vi "动态调用.vi"() -> ()   [LabVIEW 2011]
panel:
  in  "Stop Button":bool
  in  "Play Button":bool
  out "Gauge":dbl(knob) scale=0.0..10.0
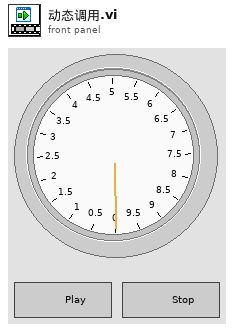
[diagram p1: front panel]
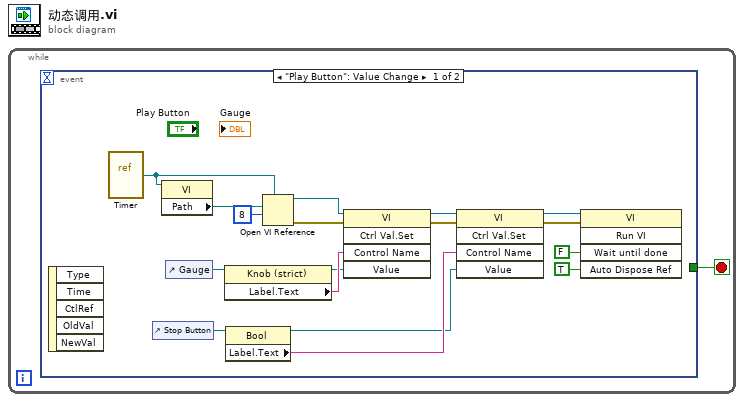
[diagram p0: block diagram]
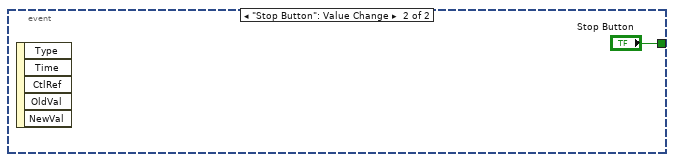
[diagram p2: hidden frame]
diagram:
  n1 = while {
    stop <- w1 stop-if-true
    n2 = event shown="[0] \"Play Button\": Value Change" {
      selector: _ -> [_ _]
      dyn-events: _ -> [_ _]
      timeout: _ -> [_ _]
      tunnel: [_ "Stop Button"] -> w1
      event "Play Button": Value Change {
        n3 = event-data() -> ()  [unwired: 1 in, 5 out]
        n4 = vi-ref "Timer.vi"() -> (w18:refnum<vi>)
        n5 = control-ref of="Stop Button"() -> (w4:refnum<vi>)
        n6 = property class="VI"(reference=w18) -> ("Path"=w17:path)  [unwired: 1 in, 2 out]
        n7 = control-ref of="Gauge"() -> (w7:refnum<vi>)
        n8 = property class="Knob (strict)"(reference=w7) -> (reference out=w5:refnum<vi>, "Label.Text"=w6:string)  [unwired: 1 in, 1 out]
        n9 = property class="Bool"(reference=w4) -> (reference out=w2:refnum<vi>, "Label.Text"=w3:string)  [unwired: 1 in, 1 out]
        n10 = Open VI Reference(type specifier VI Refnum (for type only)=w18, vi path=w17, options=8) -> (vi reference=w15:refnum<vi>, error out=w12:errorcluster)  [unwired: 3 in]
        n11 = invoke class="VI" method="Ctrl Val.Set"(reference=w15, error in=w12, "Control Name"=w6, "Value"=w5) -> (reference out=w14:refnum<vi>, error out=w11:errorcluster)  [unwired: 1 in, 3 out]
        n12 = invoke class="VI" method="Ctrl Val.Set"(reference=w14, error in=w11, "Control Name"=w3, "Value"=w2) -> (reference out=w13:refnum<vi>, error out=w10:errorcluster)  [unwired: 1 in, 3 out]
        n13 = invoke class="VI" method="Run VI"(reference=w13, error in=w10, "Wait until done"=FALSE ("Wait Until Done"), "Auto Dispose Ref"=TRUE ("Auto Dispose Reference")) -> ()  [unwired: 1 in, 5 out]
      }
      event "Stop Button": Value Change {
        n14 = event-data() -> ()  [unwired: 1 in, 5 out]
      }
    }
  }
